vi "classes.vi"(0 "HGF_DSCFactory":refnum<class "HGF_DSCFactory.lvclass">, 1 "className":string, 5 "error in (no error)":errorcluster) -> (14 "HGF_DSCFactory":refnum<class "HGF_DSCFactory.lvclass">, 16 "Object":refnum<class>, 19 "error out":errorcluster)   [LabVIEW 2012, in "HGF_DSC.lvlib" / "HGF_DSCFactory.lvclass"]
doc: "This dynamaic dispatch VI contains constant objects of all classes that can be produced by HGF_Factory.\n\nChild classes have to override it to define additional classes."
uses:
  HGF_DSCFactory.lvclass
  HGF_SV/HGF_SVFactory/HGF_SVFactory.lvclass
  HGF_DSCEvent/HGF_DSCEvent.lvclass
  HGF_DSCCommand/HGF_DSCCommand.lvclass
  HGF_DSCService/HGF_DSCService.lvclass
  HGF_DSCSubscriber/HGF_DSCSubscriber.lvclass
  HGF_DSCMonitor/HGF_DSCMonitor.lvclass
  HGF_DSCVarManager/HGF_DSCVarManager.lvclass
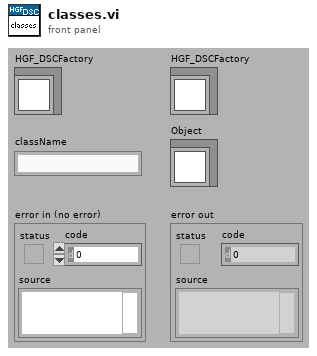
[diagram p1: front panel]
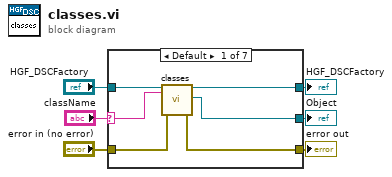
[diagram p0: block diagram]
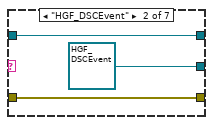
[diagram p2: hidden frame]
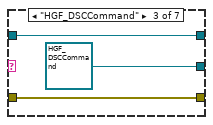
[diagram p3: hidden frame]
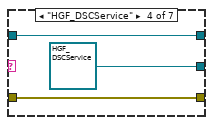
[diagram p4: hidden frame]
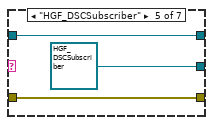
[diagram p5: hidden frame]
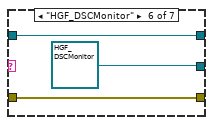
[diagram p6: hidden frame]
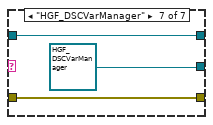
[diagram p7: hidden frame]
diagram:
  n1 = case shown="Default" "className" {
    selector: "className" -> [w7 _ _ _ _ _ _]
    tunnel: "HGF_DSCFactory" -> [w12 w13 w17 w20 w23 w26 w29]
    tunnel: "error in (no error)" -> [w11 w14 w16 w19 w22 w25 w28]
    tunnel: [w10 w13 w17 w20 w23 w26 w29] -> w4
    tunnel: [w9 refnum<class "HGF_DSCEvent.lvclass"> refnum ("DSC.lvlib:HGF_DSCEvent.lvclass") refnum<class "HGF_DSCCommand.lvclass"> refnum ("DSC.lvlib:HGF_DSCCommand.lvclass") refnum<class "HGF_DSCService.lvclass"> refnum ("DSC.lvlib:HGF_DSCService.lvclass") refnum<class "HGF_DSCSubscriber.lvclass"> refnum ("DSC.lvlib:HGF_DSCSubscriber.lvclass") refnum<class "HGF_DSCMonitor.lvclass"> refnum ("DSC.lvlib:HGF_DSCMonitor.lvclass") refnum<class "HGF_DSCVarManager.lvclass"> refnum ("DSC.lvlib:HGF_DSCVarManager.lvclass")] -> w3
    tunnel: [w8 w14 w16 w19 w22 w25 w28] -> w2
    frame Default {
      n2 = call-parent "classes.vi"("HGF_SVFactory"=w12, "className"=w7, "error in (no error)"=w11) -> ("dup HGF_SVFactory"=w10:refnum<class "HGF_DSCFactory.lvclass">, "Object"=w9:refnum<class>, "error out"=w8:errorcluster)  [unwired: 14 out]
    }
    frame "HGF_DSCEvent" {
    }
    frame "HGF_DSCCommand" {
    }
    frame "HGF_DSCService" {
    }
    frame "HGF_DSCSubscriber" {
    }
    frame "HGF_DSCMonitor" {
    }
    frame "HGF_DSCVarManager" {
    }
  }
  "error out" <- w2
  "HGF_DSCFactory" <- w4
  "Object" <- w3
